vi "punto2.vi"() -> ()   [LabVIEW 2021]
panel:
  out "Waveform Graph":dynamicdata(graph)
  in  "Generated voltage":dbl(knob) scale=0.0..5.0
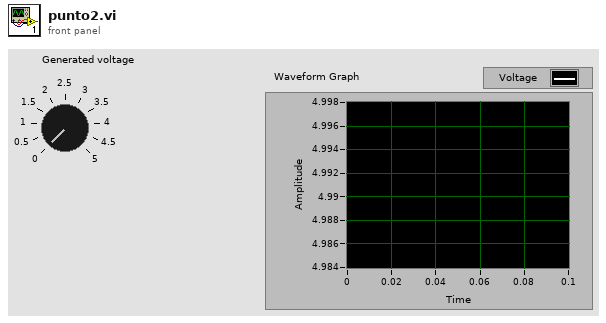
[diagram p1: front panel]
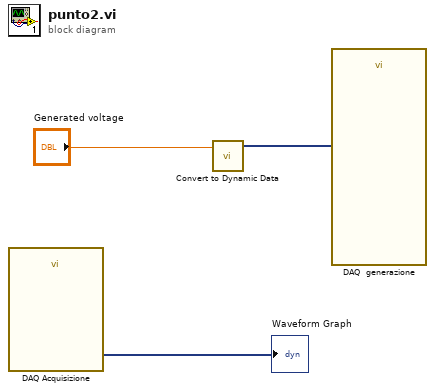
[diagram p0: block diagram]
diagram:
  n1 = call "DAQ Acquisizione"() -> ("data"=→"Waveform Graph":dynamicdata)  [unwired: 17 in, 2 out]
  n2 = call "Convert to Dynamic Data"("Double"="Generated voltage") -> ("Dynamic Data Type"=w2:dynamicdata)  [unwired: 3 in]
  n3 = call "DAQ  generazione"("data"=w2) -> ()  [unwired: 17 in, 2 out]
